vi "Analyze Image.vi"(8 "error in (no error)":errorcluster, 9 "Image Nr.":i32, 10 "Pre Procesed Image":T1, 11 "HIJ Vision Application in":refnum<class "HIJ Vision Application.lvclass">) -> (0 "error out":errorcluster, 3 "HIJ Vision Application out":refnum<class "HIJ Vision Application.lvclass">)   [LabVIEW 2020, in "HIJ Vision Application.lvlib" / "HIJ Vision Application.lvclass"]
uses:
  HIJ Vision Application.lvclass
  <vilib>/vision/Image Controls.llb/IMAQ Image.ctl
  Display Actors/HIJ Vision Display/HIJ Vision Display/Analyze.ctl
  Analyze/Analyze Classes/Analyze BaseClass/Analyze BaseClass/Analyze BaseClass.lvclass
  Analyze/Results and Overlays/Results Base/Analyze Results Base.lvclass
  HIJ Vision Application.lvclass/HIJ Vision Application.ctl
  Analyze/Analyze Actor/Analyze Actor Messages/Analyze Msg/Analyze Msg.lvclass/Analyze Msg.ctl
  <vilib>/ActorFramework/Message Enqueuer/Message Enqueuer.lvclass/Message Enqueuer.ctl
  <vilib>/ActorFramework/Message Enqueuer/Enqueue.vi
  Analyze/Analyze Actor/Analyze Actor Messages/Analyze Msg/Analyze Msg.lvclass
  C:/Program Files (x86)/National Instruments/LabVIEW 2020/vi.lib/ActorFramework/Message/Message.lvclass
  <vilib>/ActorFramework/Message Priority Queue/Priority Enqueue.vi
  Analyze/Analyze Actor/Analyze Actor/Analyze Actor.lvclass
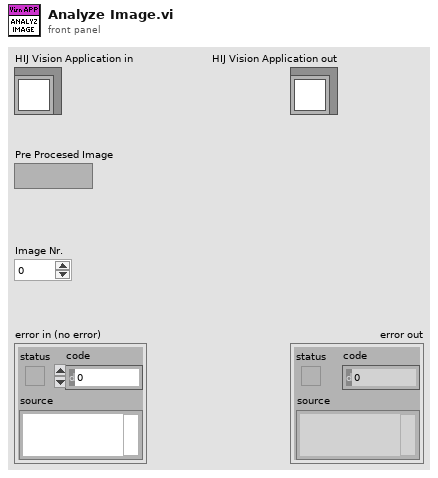
[diagram p1: front panel]
types:
  T1 = typedef "IMAQ Image.ctl" = refnum<image>
  T2 = typedef "Analyze Actor.lvlib/Analyze Actor.lvclass/Analyze.ctl" = cluster{"Image":T1, "ImageNr":i32, "Analyze Objects":refnum<class "Analyze BaseClass.lvclass">[], "Pre Results":refnum<class "Analyze Results Base.lvclass">[]}
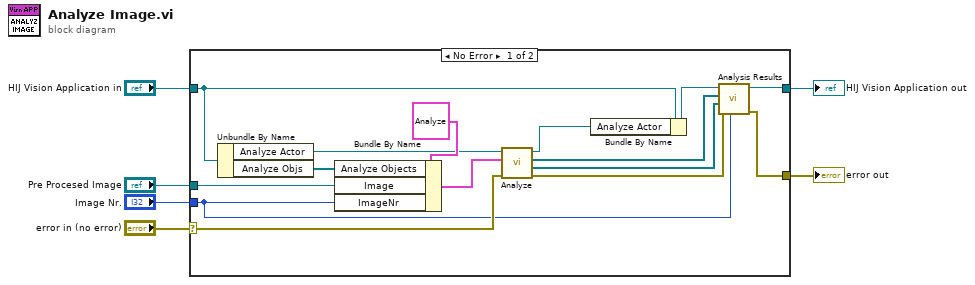
[diagram p0: block diagram]
diagram:
  n1 = case shown="No Error" "error in (no error)" {
    selector: "error in (no error)" -> [w16 w23]
    tunnel: [w10 w23] -> w5
    tunnel: [w12 w22] -> w3
    tunnel: "HIJ Vision Application in" -> [w11 w22]
    tunnel: "Pre Procesed Image" -> [w20 _]
    tunnel: "Image Nr." -> [w9 _]
    frame No Error {
      n2 = Unbundle By Name(w11) -> ("Analyze Actor"=w18:refnum<class "Analyze Actor.lvclass">, "Analyze Objs"=w19:refnum<class "Analyze BaseClass.lvclass">[])
      n3 = Bundle By Name(cluster=T2 {"Image"=refnum, "ImageNr"=0, "Analyze Objects"=[], "Pre Results"=[]} ("Analyze data"), "Analyze Objects"=w19, "Image"=w20, "ImageNr"=w9) -> (w17:T2)
      n4 = call-dynamic "Analyze.vi"("error in (no error)"=w16, "Analyze Data"=w17, "Analyze Actor.lvlib:Analyze Actor.lvclass"=w18) -> ("error out"=w13:errorcluster, "Results"=w14:refnum<class "Analyze Results Base.lvclass">[], "Parameters"=w15:refnum<class "Analyze Parameter Base.lvclass">[], "Analyze Actor.lvlib:Analyze Acto out"=w7:refnum<class "Analyze Actor.lvclass">)  [unwired: 5 in]
      n5 = Bundle By Name(cluster=w11, "Analyze Actor"=w7) -> (w8:refnum<class "HIJ Vision Application.lvclass">)
      n6 = call-dynamic "Analysis Results.vi"("Image Nr."=w9, "error in (no error)"=w13, "Results In"=w14, "Parameters"=w15, "Launch IMAQ Display in"=w8) -> ("error out"=w10:errorcluster, "Launch IMAQ Display out"=w12:refnum<class "HIJ Vision Application.lvclass">)  [unwired: 5 in]
    }
    frame Error {
    }
  }
  "error out" <- w5
  "HIJ Vision Application out" <- w3
